vi "Main On Compile Action VI.vi"(8 "error in (no error)":errorcluster, 11 "Device Item Ref in":T1 format="%.0x") -> (0 "error out":errorcluster)   [LabVIEW 2014, in "SLSC configuration System Explorer.lvlib"]
uses:
  SLSC configuration System Explorer.lvlib
  <vilib>/NI Veristand/Custom Device API/Custom Device Item Ref.ctl
  Shared/Type Defs/SLSC compiled.ctl
  Shared/Type Defs/Res Sim compiled.ctl
  Shared/Type Defs/RT Engine Data.ctl
  Shared/Type Defs/RT IDs.ctl
  Shared/SPI Utility/Slot #.ctl
  Shared/MCP23S17/Chip Address.ctl
  Shared/Constants.vi
  <vilib>/NI Veristand/Custom Device API/Set Item Property (Variant).vi
  <vilib>/NI Veristand/Custom Device API/Custom Device API.lvlib
  Shared/SLSC configuration Shared.lvlib
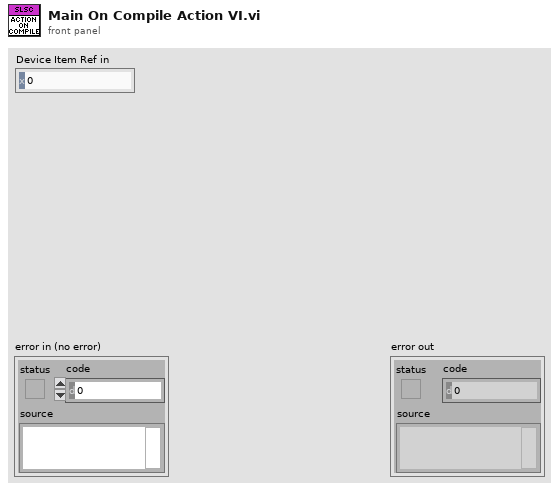
[diagram p1: front panel]
types:
  T1 = typedef "Custom Device API.lvlib/Custom Device Item Ref.ctl" = u64
  T2 = typedef "SLSC configuration Shared.lvlib/SLSC compiled.ctl" = cluster{"Initial SPI CMDs":u64[], "Res Sim data ":T3[], "Res Sim init FIFO elements":u32[], "FIU Engine Data":T4, "Battery Switch Engine Data":T4, "Wheel Speed Sensor Engine Data":T4, "Resistor Engine Data":T4, "Current Sense Engine Data":T4}
  T3 = typedef "SLSC configuration Shared.lvlib/Res Sim compiled.ctl" = cluster{"FIFO bytes3_2":u16, "Channel Old Value":dbl, "Channel data ref":i32}
  T4 = typedef "SLSC configuration Shared.lvlib/RT Engine Data.ctl" = cluster{"RT IDs":T5[], "Ordered Channels":T1[]}
  T5 = typedef "SLSC configuration Shared.lvlib/RT IDs.ctl" = cluster{"Rack #":u8, "Slot #":T6, "Chip Address (A2 A1 A0)":T7}
  T6 = typedef "SLSC configuration Shared.lvlib/Slot #.ctl" = u8
  T7 = typedef "SLSC configuration Shared.lvlib/Chip Address.ctl" = u8
  T8 = typedef "SLSC configuration Shared.lvlib/Device Settings.ctl" = cluster{"RIO Address":string, "Bitfile Path":path, "Load Delay (ms)":u32, "Divide Value":u8, "Sample Rate (S/s)":u32, "SLSC Settings":string, "SLSC FIFO Name":string}
  T9 = typedef "SLSC configuration Shared.lvlib/UEGO Compile Info.ctl" = cluster{"FPGA Item Name":string, "UEGOcalibration.<user name>":T10}
  T10 = typedef "SLSC FPGA Toolkit.lvlib/SLSC UEGO Calibration.ctl" = cluster{"Rack #":u8, "CS Bit Value/Slot #":u8, "Calibration Ticks":u32, "HW Settling Ticks":u32}
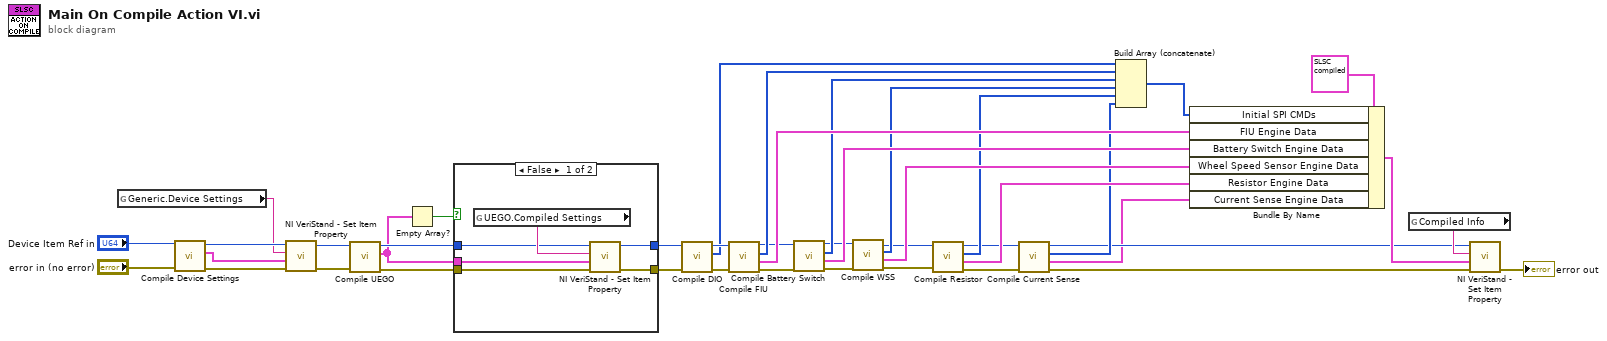
[diagram p0: block diagram]
diagram:
  n1 = global read "Constants.vi" "Generic.Device Settings"() -> (w34:string)
  n2 = call "Compile Device Settings.vi"("error in (no error)"="error in (no error)", "Device Ref in"="Device Item Ref in") -> ("error out"=w36:errorcluster, "Device Settings"=w15:T8, "Device Ref out"=w35:T1)  [unwired: 7 in]
  n3 = call-poly <vilib>:"NI VeriStand - Set Item Property.vi"("error in (no error)"=w36, "Value"=w15, "Property Name"=w34, "Item Ref in"=w35) -> ("error out"=w14:errorcluster, "Item Ref out"=w13:T1)  [unwired: 5 in, 1 out]
  n4 = call "Compile UEGO.vi"("error in (no error)"=w14, "Device Ref in"=w13) -> ("error out"=w12:errorcluster, "UEGO Calibration Info"=w8:T9[], "Device Ref out"=w9:T1)  [unwired: 7 in]
  n5 = Empty Array?(array=w8) -> (empty?=w7:bool)
  n6 = case shown="False" w7 {
    tunnel: w12 -> [w47 w49]
    tunnel: [w46 w49] -> w11
    tunnel: [w45 w50] -> w10
    tunnel: w9 -> [w44 w50]
    tunnel: w8 -> [w43 _]
    frame False {
      n7 = global read "Constants.vi" "UEGO.Compiled Settings"() -> (w48:string)
      n8 = call-poly <vilib>:"NI VeriStand - Set Item Property.vi"("error in (no error)"=w47, "Value"=w43, "Property Name"=w48, "Item Ref in"=w44) -> ("error out"=w46:errorcluster, "Item Ref out"=w45:T1)  [unwired: 5 in, 1 out]
    }
    frame True {
    }
  }
  n9 = call "Compile DIO.vi"("error in (no error)"=w11, "Device Item Ref in"=w10) -> ("error out"=w40:errorcluster, "Initial DIO SPI CMDs"=w31:u64[], "Device Item Ref out"=w39:T1)  [unwired: 7 in]
  n10 = call "Compile FIU.vi"("error in (no error)"=w40, "Device Item Ref in"=w39) -> ("error out"=w27:errorcluster, "FIU Engine Data"=w28:T4, "Initial FIU SPI CMDs"=w30:u64[], "Device Item Ref out"=w26:T1)  [unwired: 6 in]
  n11 = call "Compile Battery Switch.vi"("error in (no error)"=w27, "Device Item Ref in"=w26) -> ("error out"=w23:errorcluster, "Battery Switch Engine Data"=w24:T4, "Initial Battery Switch SPI CMDs"=w25:u64[], "Device Item Ref out"=w22:T1)  [unwired: 6 in]
  n12 = call "Compile WSS.vi"("error in (no error)"=w23, "Device Item Ref in"=w22) -> ("error out"=w19:errorcluster, "Wheel Speed Sensor Engine Data"=w20:T4, "Initial Wheel Speed Sensor SPI CMDs"=w21:u64[], "Device Item Ref out"=w18:T1)  [unwired: 6 in]
  n13 = call "Compile Resistor.vi"("error in (no error)"=w19, "Device Item Ref in"=w18) -> ("error out"=w6:errorcluster, "Resistor Engine Data"=w16:T4, "Initial Resistor SPI CMDs"=w17:u64[], "Device Item Ref out"=w5:T1)  [unwired: 6 in]
  n14 = call "Compile Current Sense.vi"("error in (no error)"=w6, "Device Item Ref in"=w5) -> ("error out"=w2:errorcluster, "Wheel Speed Sensor Engine Data"=w1:T4, "Initial Wheel Speed Sensor SPI CMDs"=w4:u64[], "Device Item Ref out"=w3:T1)  [unwired: 6 in]
  n15 = Build Array (concatenate)(w31, w30, w25, w21, w17, w4) -> (w29:u64[])
  n16 = Bundle By Name(cluster=T2 {"Initial SPI CMDs"=[], "Res Sim data "=[], "Res Sim init FIFO elements"=[], "FIU Engine Data"={"RT IDs"=[], "Ordered Channels"=[]}, "Battery Switch Engine Data"={"RT IDs"=[], "Ordered Channels"=[]}, "Wheel Speed Sensor Engine Data"={"RT IDs"=[], "Ordered Channels"=[]}, "Resistor Engine Data"={"RT IDs"=[], "Ordered Channels"=[]}, "Current Sense Engine Data"={"RT IDs"=[], "Ordered Channels"=[]}} ("SLSC Compiled out"), "Initial SPI CMDs"=w29, "FIU Engine Data"=w28, "Battery Switch Engine Data"=w24, "Wheel Speed Sensor Engine Data"=w20, "Resistor Engine Data"=w16, "Current Sense Engine Data"=w1) -> (w32:T2)
  n17 = global read "Constants.vi" "Compiled Info"() -> (w42:string)
  n18 = call-poly <vilib>:"NI VeriStand - Set Item Property.vi"("error in (no error)"=w2, "Value"=w32, "Property Name"=w42, "Item Ref in"=w3) -> ("error out"=→"error out":errorcluster)  [unwired: 5 in, 2 out]
